vi "Read UI Setting.vi"(8 "error in (no error)":errorcluster, 11 "File Path":path=path "D:/GitHub/UI-Frame/UI Setting.ini") -> (0 "error out":errorcluster, 3 "Module Definition":T1[](array[typedef]))   [LabVIEW 2020, in "Group Interface.lvlib"]
uses:
  Group Interface.lvlib
  Module Definition--cluster.ctl
  Function Item--cluster.ctl
  <vilib>/Utility/config.llb/Read Key (String).vi
  <vilib>/Utility/config.llb/NI_LVConfig.lvlib
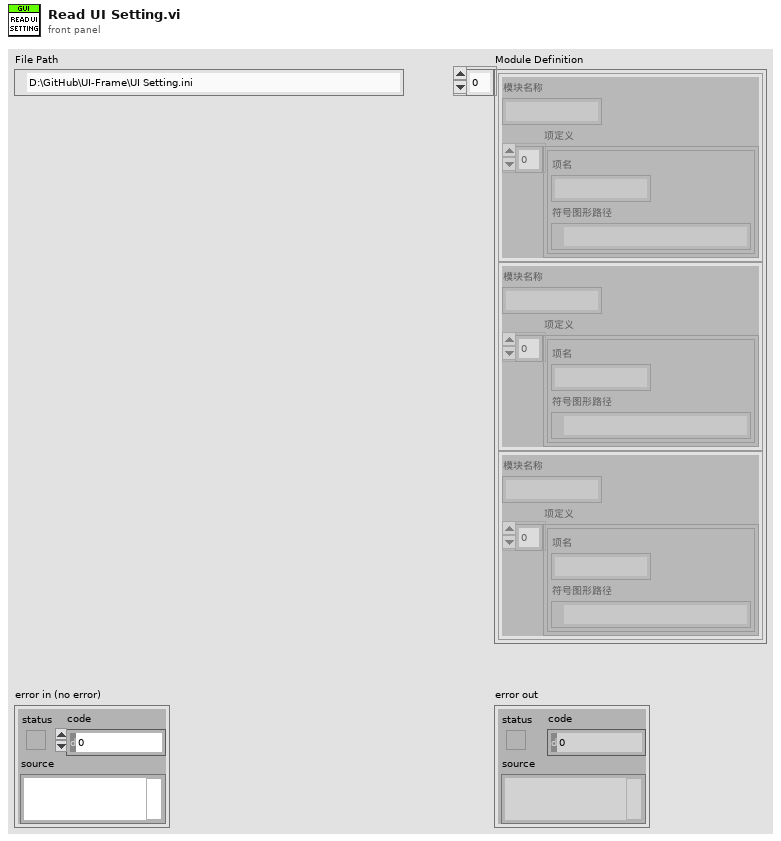
[diagram p1: front panel]
types:
  T1 = typedef "Group Interface.lvlib/Module Definition--cluster.ctl" = cluster{"模块名称":string, "项定义":T2[]}
  T2 = typedef "Group Interface.lvlib/Function Item--cluster.ctl" = cluster{"项名":string, "符号图形路径":path}
  T3 = typedef "NI_LVConfig.lvlib/Config Data RefNum.ctl" = refnum<k1>
  T4 = cluster{"String":string, cluster{"String":string, "value":string}[]}
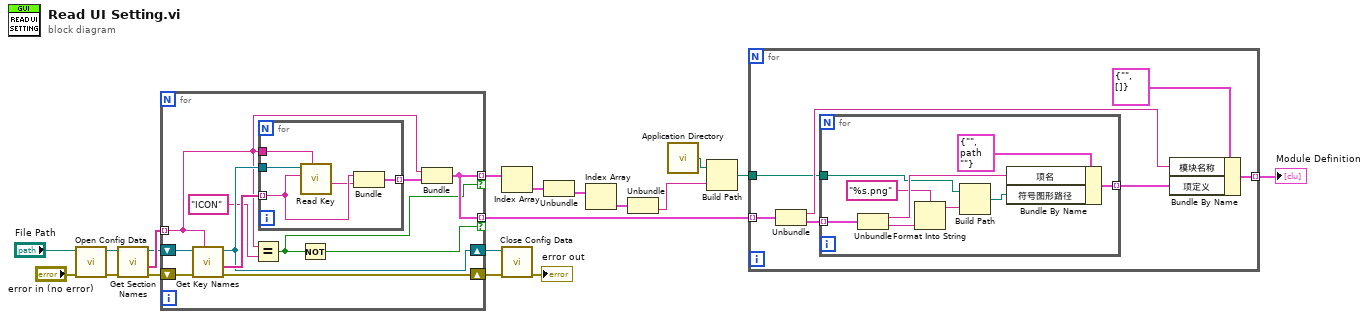
[diagram p0: block diagram]
diagram:
  n1 = call <vilib>:"Open Config Data.vi"("error in (no error)"="error in (no error)", "configuration file path"="File Path") -> ("error out"=w17:errorcluster, "refnum"=w18:T3)  [unwired: 7 in, 1 out]
  n2 = call <vilib>:"Get Section Names.vi"("error in (no error)"=w17, "refnum"=w18) -> ("error out"=w14:errorcluster, "section names"=w16:string[], "refnum out"=w15:T3)  [unwired: 7 in]
  n3 = for {
    tunnel: w16 -> [w24] mode=indexing
    tunnel: [w21] -> w5 mode=indexing if=w22
    shift-right: [w25] -> w13
    shift-left: w15 -> [w30]
    shift-right: [w26] -> w12
    shift-left: w14 -> [w27]
    tunnel: [w21] -> w11 mode=indexing if=w20
    n4 = call <vilib>:"Get Key Names.vi"("section"=w24, "error in (no error)"=w27, "refnum"=w30) -> ("error out"=w26:errorcluster, "key names"=w29:string[], "refnum out"=w25:T3)  [unwired: 5 in, 1 out]
    n5 = Equal?(x=w24, y="ICON") -> (x = y?=w20:bool)
    n6 = for {
      tunnel: w24 -> [w35]
      tunnel: w29 -> [w34] mode=indexing
      tunnel: [w32] -> w28 mode=indexing
      tunnel: w25 -> [w31]
      n7 = call-poly <vilib>:"Read Key.vi"("section"=w35, "key"=w34, "refnum"=w31) -> ("value"=w33:string)  [unwired: 5 in, 3 out]
      n8 = Bundle("String"=w34, "value"=w33) -> (w32:cluster{"String":string, "value":string})  [unwired: 1 in]
    }
    n9 = Not(x=w20) -> (.not. x?=w22:bool)
    n10 = Bundle("String"=w24, w28) -> (w21:T4)  [unwired: 1 in]
  }
  n11 = Index Array(array=w11) -> (element=w10:T4)  [unwired: 1 in]
  n12 = call <vilib>:"Close Config Data.vi"("error in (no error)"=w12, "refnum"=w13) -> ("error out"=→"error out":errorcluster)  [unwired: 8 in, 1 out]
  n13 = Unbundle(w10) -> (w9:cluster{"String":string, "value":string}[])  [unwired: 1 out]
  n14 = Index Array(array=w9) -> (element=w8:cluster{"String":string, "value":string})  [unwired: 1 in]
  n15 = Unbundle(w8) -> ("value"=w6:string)  [unwired: 1 out]
  n16 = call <vilib>:"Application Directory.vi"() -> ("Application Directory"=w7:path)
  n17 = Build Path(base path=w7, name or relative path=w6) -> (appended path=w3:path)
  n18 = for {
    tunnel: w5 -> [w42] mode=indexing
    tunnel: [w37] -> w4 mode=indexing
    tunnel: w3 -> [w36]
    n19 = Unbundle(w42) -> ("String"=w40:string, w39:cluster{"String":string, "value":string}[])
    n20 = for {
      tunnel: w39 -> [w51] mode=indexing
      tunnel: [w48] -> w38 mode=indexing
      tunnel: w36 -> [w47]
      n21 = Unbundle(w51) -> ("String"=w49:string, "value"=w46:string)
      n22 = Format Into String(format string="%s.png", w46) -> (resulting string=w44:string)  [unwired: 2 in, 1 out]
      n23 = Build Path(base path=w47, name or relative path=w44) -> (appended path=w43:path)
      n24 = Bundle By Name(cluster=T2 {"项名"="", "符号图形路径"=path ""} ("簇"), "项名"=w49, "符号图形路径"=w43) -> (w48:T2)
    }
    n25 = Bundle By Name(cluster=T1 {"模块名称"="", "项定义"=[]} ("模块定义"), "模块名称"=w40, "项定义"=w38) -> (w37:T1)
  }
  "Module Definition" <- w4
